vi "DunkFlips.vi"() -> ()   [LabVIEW 2015]
uses:
  <vilib>/Platform/TimedLoop/XDataNode/timing_clust.ctl
  <vilib>/Platform/TimedLoop/XDataNode/nitl_modes.ctl
  <vilib>/Platform/TimedLoop/XDataNode/wakeup.ctl
  <vilib>/rvi/Emulation/niFpgaGetClockAttributes.vi
  <vilib>/rvi/Emulation/niFpgaSctlEmulationGetInTimedLoop.vi
  <vilib>/rvi/Emulation/niFpgaEmulationReportErrorSimple.vi
  <vilib>/rvi/DataTransferAndStorage/Container/Common/niFpgaContainerGetUniqueNameForEmu.vi
  <vilib>/rvi/DataTransferAndStorage/Container/Common/niFpgaContainerSetEmuInfo.vi
  <vilib>/rvi/eio/common/nirviEmuReportErrorAndStop.vi
  <vilib>/rvi/eio/common/nirviEmuTemplateMethod_errors.vi
  <vilib>/rvi/DataTransferAndStorage/Container/Common/niFpgaContainerExecOnDevCompGetState.vi
  <vilib>/rvi/Emulation/niFpgaEmulationIsFPGAContextNoSignature.vi
  <vilib>/rvi/errors/niFpgaSetErrorForExecOnDevCompSimple.vi
  <vilib>/rvi/FIFO/Fifo_Resource/nirvififoEmulationSetSize.vi
  <vilib>/rvi/FIFO/Fifo_Resource/nirviFifoEmulationQueueMgr.vi
  <instcachedir>/0/nirviFifoEmulationQueueMgr_E5CAEC123FF24DC58D834DCA3CDAA9B5.lvgen/nirviFifoEmulationQueueMgr_E5CAEC123FF24DC58D834DCA3CDAA9B5_001.vi
  <vilib>/rvi/FIFO/Fifo_Resource/nirvififoEmulationDetermineInputValidOut.vi
  <vilib>/rvi/FIFO/Fifo_Resource/nirvififoEmulationCreateLock.vi
  <vilib>/rvi/Emulation/niFpgaProcessEmulError.vi
  <vilib>/rvi/FIFO/Fifo_Resource/nirvififoEmulationObtainLock.vi
  <vilib>/rvi/FIFO/Fifo_Resource/nirvififoEmulationReleaseLock.vi
  <vilib>/rvi/occurrence/nirviWaitOnOccurrenceBase.vi
  <vilib>/rvi/errors/nirviReportUnexpectedCaseInternalError.vi
  <vilib>/rvi/errors/nirviReportUnexpectedCaseInternalError (U32).vi
  <vilib>/Utility/error.llb/Clear Errors.vi
  <vilib>/rvi/interface/RandomDataEmulation/niFpgaRandomDataHandleErrors.vi
  <vilib>/rvi/Emulation/niFpgaCriticalErrorInLSC.vi
  <vilib>/rvi/Analysis/common/codeGenErrors/XNode/niFpgaXNodeCodeGenErrorHandle.vi
  <vilib>/rvi/Analysis/utilities/niFPGA Threshold Crossing Logic.vi
  <instcachedir>/0/nirviFifoEmulationQueueMgr_E5CAEC123FF24DC58D834DCA3CDAA9B5.lvgen/nirviFifoEmulationQueueMgr_E5CAEC123FF24DC58D834DCA3CDAA9B5_004.vi
  <instcachedir>/0/nirviFifoEmulationQueueMgr_E5CAEC123FF24DC58D834DCA3CDAA9B5.lvgen/nirviFifoEmulationQueueMgr_E5CAEC123FF24DC58D834DCA3CDAA9B5_000.vi
  <vilib>/rvi/LocalResourceManager/LocalResourceManager.xnode
  <vilib>/eio/EIONode/EIONode.xnode
  <vilib>/rvi/DataTransferAndStorage/Container/XNode/niFpgaContainer.xnode
  <vilib>/rvi/FIFO/Fifo_Resource/niFpgaFifoEmulationRefIn.vi
  <vilib>/rvi/Analysis/measure/period/templates/niFPGA Period Edge Direction.ctl
  <vilib>/rvi/Analysis/measure/butterworth/XNode/niFpgaButterworthFilter.xnode
  <vilib>/rvi/Analysis/measure/period/XNode/niFpgaAnalogPeriod.xnode
  <vilib>/Platform/TimedLoop/XDataNode/XDataNode.xnode
  <vilib>/rvi/FXPMathLib/basic elements/FxpDiscreteDelay/XNode/nifxpmath_DiscreteDelay.xnode
  <vilib>/rvi/interface/RandomDataEmulation/nirviRandomDataFpgaReadWriteTemplate.vi
  <vilib>/Platform/TimedLoop/XDataNode/XDNodeRunTimeDep.lvlib
panel:
  out "Time":i64=15
  out "TDOA 3":i64
  out "TDOA 2":i64
  out "TDOA 1":i64
  out "Period 4":u32=17
  out "Period 3":u32=15
  out "Period 1":u32=14
  out "Period 2":u32=30
  out "Boolean 4":bool
  out "Boolean 3":bool
  out "Boolean 2":bool
  out "Boolean":bool
  out "unsigned value":u16=109
  out "byte value":u16
  out "qfgLO!":i16=109
  in  "Baud Rate":u32=9600
  out "Real Baud Rate":u32=4167
  out "Des BABaus":u32=4167
  out "DIO Max":u16=18
  out "DIO Min":u16=15
  in  "FIFO Signal":u32
  out "Output 3":i64
  in  "High Pass":bool=TRUE
  in  "Low Pass":bool=TRUE
  in  "Hysteresis 4":fxp<+,16,2>
  in  "Hysteresis 3":fxp<+,16,2>
  in  "Hysteresis 2":fxp<+,16,2>
  out "Actual Sample Period Process (ticks)":u32=80
  in  "Min signal time gap (samples)":u32=500000
  in  "Min Amplitude 1":fxp<+/-,16,3>=0.0050048828125
  out "Output 1":i64
  out "AI0":sgl(slide)=-0.00048828125 scale=-10.0..10.0
  in  "Min Amplitude 2":fxp<+/-,16,3>=0.0050048828125
  out "Output 2":i64
  out "AI1":sgl(slide) scale=-10.0..10.0
  in  "Min Amplitude 3":fxp<+/-,16,3>=0.0050048828125
  out "AI2":sgl(slide)=-0.00048828125 scale=-10.0..10.0
  out "Output 4":i64
  in  "Hysteresis 1":fxp<+,16,2>
  in  "Min Amplitude 4":fxp<+/-,16,3>=0.0050048828125
  out "AI3":sgl(slide)=0.00024414062 scale=-10.0..10.0
  in  "Requested Sample Period (ticks)":u32=80
  out "Actual Sample Period Wave (ticks)":u32=80
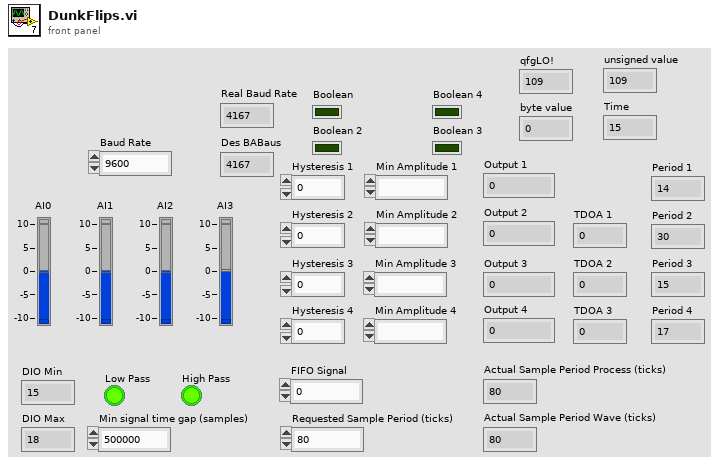
[diagram p1: front panel]
types:
  T1 = typedef "XDNodeRunTimeDep.lvlib/timing_clust.ctl" = cluster{"Expected End [f-1]":u64, "Actual End [f-1]":u64, "Finished Late? [f-1]":bool, "Expected End [i-1]":u64, "Actual End [i-1]":u64, "Finished Late? [i-1]":bool, "Expected Start [i]":u64, "Actual Start [i]":u64, "Expected Start [f]":u64, "Actual Start [f]":u64, "Source Name":string, "Structure Name":string, "Period":i64, "Deadline":i64, "Offset":i64, "Start":i64, "Priority":i32, "Timeout":i32, "Mode":T2, "Wakeup Reason":T3, "Error":errorcluster, "Source Type":string, "Secondary Source Type":string, "Global End Time":u64, "Global Start Time":u64, "Frame Duration":u64, "Iteration Duration":u64, "Assigned CPU":i32, "I/O Scan Engine Mode":u32}
  T2 = typedef "XDNodeRunTimeDep.lvlib/nitl_modes.ctl" = enum32{"No Change", "Process missed periods, maintain original phase", "Discard missed periods, maintain original phase", "Process missed periods, ignore original phase", "Discard missed periods, ignore original phase"}
  T3 = typedef "XDNodeRunTimeDep.lvlib/wakeup.ctl" = enum32{"Normal", "Aborted", "Asynchronous wakeup", "Timing source error", "Timed loop error", "Timeout"}
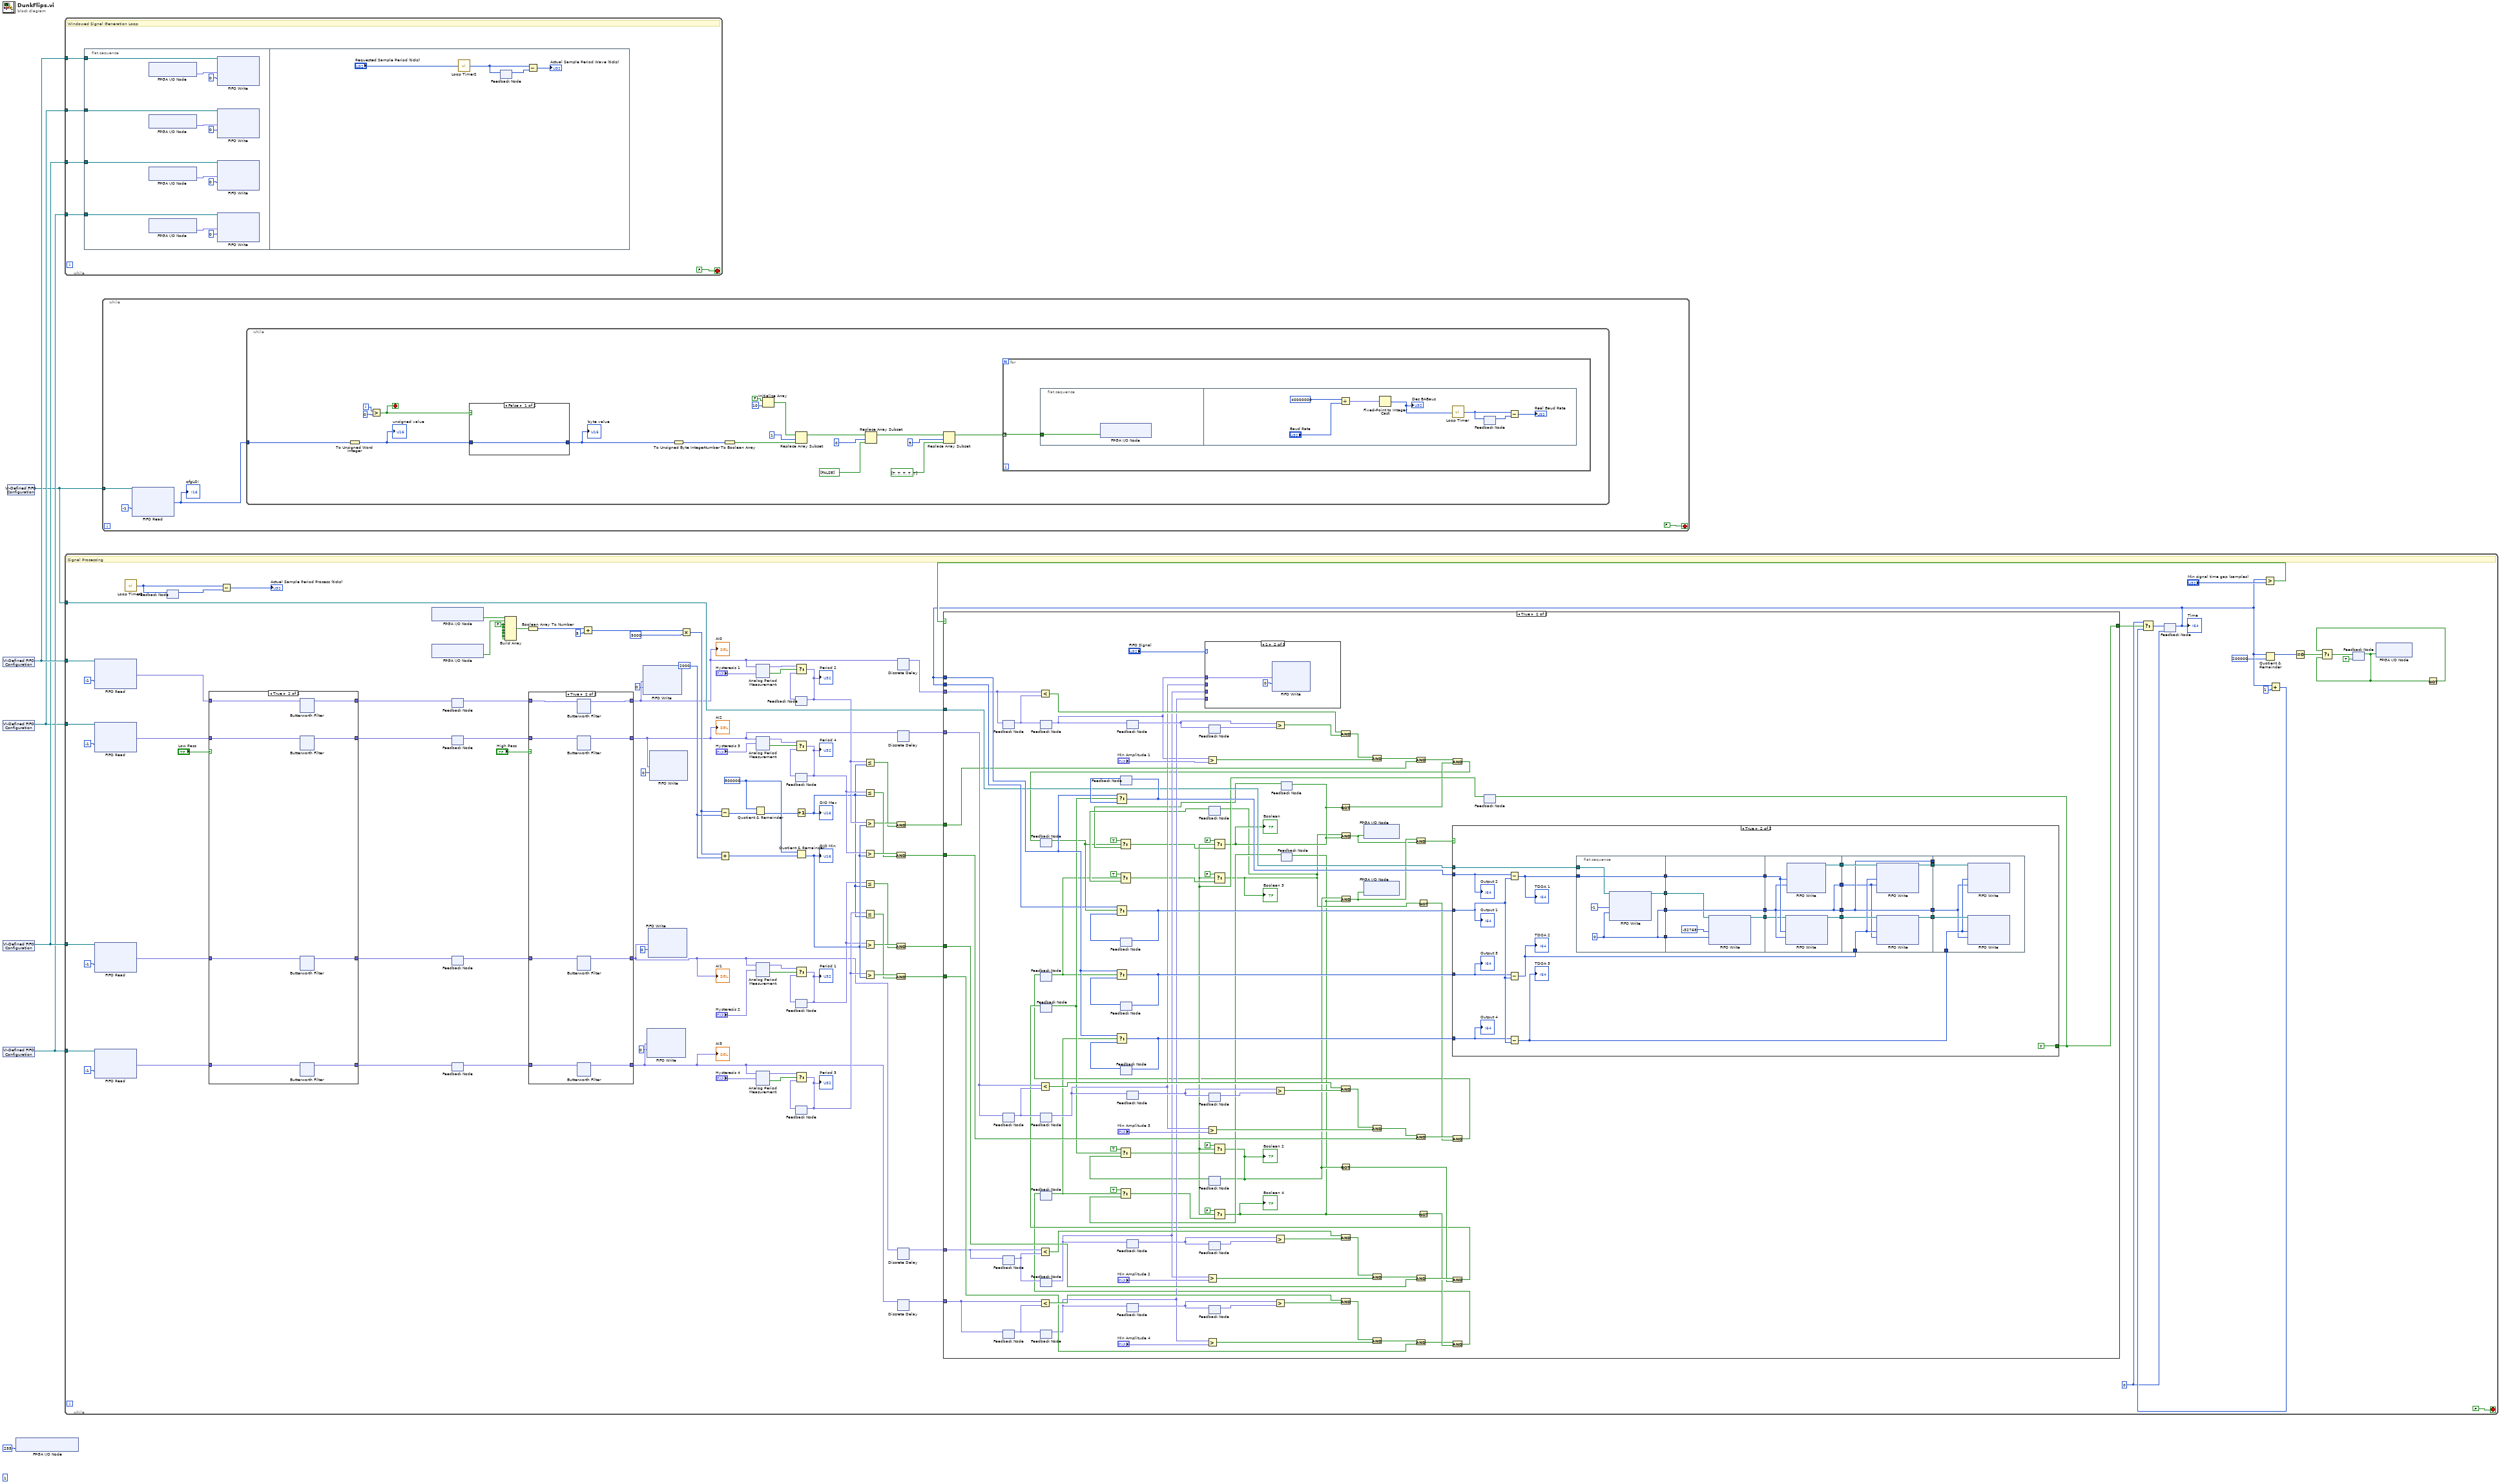
[diagram p0: block diagram]
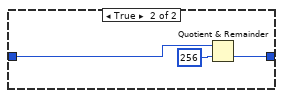
[diagram p2: hidden frame]
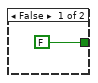
[diagram p5: hidden frame]
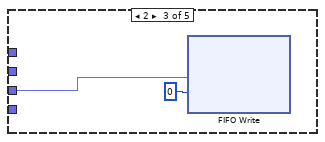
[diagram p7: hidden frame]
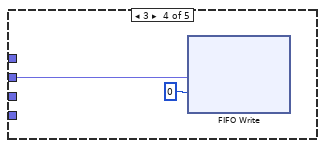
[diagram p8: hidden frame]
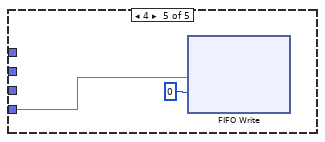
[diagram p9: hidden frame]
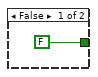
[diagram p10: hidden frame]
diagram:
  (unwired) 1 ("y")
  n1 = xnode "VI-Defined FIFO Configuration"() -> ("FIFO Out"=w6:refnum<k21>)
  n2 = xnode "VI-Defined FIFO Configuration"() -> ("FIFO Out"=w3:refnum<k21>)
  n3 = xnode "VI-Defined FIFO Configuration"() -> ("FIFO Out"=w5:refnum<k21>)
  n4 = xnode "VI-Defined FIFO Configuration"() -> ("FIFO Out"=w4:refnum<k21>)
  n5 = xnode "VI-Defined FIFO Configuration"() -> ("FIFO Out"=w2:refnum<k21>)
  n6 = xnode "FPGA I/O Node"("Connector3/DIOPORT0"=u8 255) -> ()  [unwired: 1 in, 1 out]
  n7 = while {
    tunnel: w6 -> [w11]
    tunnel: w5 -> [w9]
    tunnel: w3 -> [w8]
    tunnel: w4 -> [w7]
    stop <- FALSE stop-if-true
    # "Windowed Signal Generation Loop"
    n8 = flat-sequence {
      tunnel: w11 -> [w18]
      tunnel: w9 -> [w17]
      tunnel: w8 -> [w16]
      tunnel: w7 -> [w19]
      frame #0 {
        n9 = xnode "FPGA I/O Node"() -> ("Connector0/AI0"=w15:fxp<+/-,27,5>)  [unwired: 1 in, 1 out]
        n10 = xnode "FPGA I/O Node"() -> ("Connector0/AI2"=w13:fxp<+/-,27,5>)  [unwired: 1 in, 1 out]
        n11 = xnode "FPGA I/O Node"() -> ("Connector0/AI1"=w12:fxp<+/-,27,5>)  [unwired: 1 in, 1 out]
        n12 = xnode "FPGA I/O Node"() -> ("Connector0/AI3"=w14:fxp<+/-,27,5>)  [unwired: 1 in, 1 out]
        n13 = xnode ("FIFO Write")("Element"=w15, "Timeout"=0, "FIFO In"=w18) -> ()  [unwired: 2 out]
        n14 = xnode ("FIFO Write")("Element"=w13, "Timeout"=0, "FIFO In"=w16) -> ()  [unwired: 2 out]
        n15 = xnode ("FIFO Write")("Element"=w12, "Timeout"=0, "FIFO In"=w17) -> ()  [unwired: 2 out]
        n16 = xnode ("FIFO Write")("Element"=w14, "Timeout"=0, "FIFO In"=w19) -> ()  [unwired: 2 out]
      }
      frame #1 {
        n17 = call "Loop Timer2"("Count(Ticks)"="Requested Sample Period (ticks)") -> ("Tick Count(Ticks)"=w24:u32)
        n18 = feedback #1() -> (w25:u32)  [unwired: 1 in]
        n19 = feedback-in #1(w24) -> ()
        n20 = Subtract(x=w24, y=w25) -> (x-y=→"Actual Sample Period Wave (ticks)":u32)
      }
    }
  }
  n21 = while {
    tunnel: w6 -> [w111]
    tunnel: w5 -> [w112]
    tunnel: w3 -> [w110]
    tunnel: w4 -> [w124]
    tunnel: w2 -> [w70]
    stop <- FALSE stop-if-true
    w47 = i64 0
    w62 = u32 500000
    w66 = i16 2000
    w65 = FALSE
    # "Signal Processing"
    n22 = xnode ("FIFO Read")("Timeout"=i16 -1, "FIFO In"=w111) -> ("Element"=w90:fxp<+/-,16,4>)  [unwired: 2 out]
    n23 = xnode ("FIFO Read")("Timeout"=i16 -1, "FIFO In"=w110) -> ("Element"=w86:fxp<+/-,16,4>)  [unwired: 2 out]
    n24 = xnode ("FIFO Read")("Timeout"=i16 -1, "FIFO In"=w112) -> ("Element"=w89:fxp<+/-,16,4>)  [unwired: 2 out]
    n25 = xnode ("FIFO Read")("Timeout"=i16 -1, "FIFO In"=w124) -> ("Element"=w83:fxp<+/-,16,4>)  [unwired: 2 out]
    n26 = call "Loop Timer3"() -> ("Tick Count(Ticks)"=w103:u32)  [unwired: 1 in]
    n27 = feedback #2() -> (w104:u32)  [unwired: 1 in]
    n28 = feedback-in #2(w103) -> ()
    n29 = case shown="True" "Low Pass" {
      tunnel: [w173 w181] -> w91
      tunnel: w90 -> [w173 w180]
      tunnel: w89 -> [w172 w179]
      tunnel: [w172 w178] -> w88
      tunnel: w86 -> [w170 w177]
      tunnel: [w170 w176] -> w85
      tunnel: w83 -> [w171 w175]
      tunnel: [w171 w174] -> w82
      frame False {
      }
      frame True {
        n30 = xnode "Butterworth Filter"("input data"=w180) -> ("output data"=w181:fxp<+/-,20,8>)  [unwired: 2 in]
        n31 = xnode "Butterworth Filter"("input data"=w177) -> ("output data"=w176:fxp<+/-,20,8>)  [unwired: 2 in]
        n32 = xnode "Butterworth Filter"("input data"=w179) -> ("output data"=w178:fxp<+/-,20,8>)  [unwired: 2 in]
        n33 = xnode "Butterworth Filter"("input data"=w175) -> ("output data"=w174:fxp<+/-,20,8>)  [unwired: 2 in]
      }
    }
    n34 = Subtract(x=w103, y=w104) -> (x-y=→"Actual Sample Period Process (ticks)":u32)
    n35 = xnode "FPGA I/O Node"() -> ("Connector2/DIO0"=w69:bool)  [unwired: 1 in, 1 out]
    n36 = xnode "FPGA I/O Node"() -> ("Connector2/DIO1"=w68:bool)  [unwired: 1 in, 1 out]
    n37 = feedback #3() -> (w92:fxp<+/-,20,8>)  [unwired: 1 in]
    n38 = feedback-in #3(w91) -> ()
    n39 = feedback #4() -> (w84:fxp<+/-,20,8>)  [unwired: 1 in]
    n40 = feedback-in #4(w85) -> ()
    n41 = feedback #5() -> (w87:fxp<+/-,20,8>)  [unwired: 1 in]
    n42 = feedback-in #5(w88) -> ()
    n43 = feedback #6() -> (w81:fxp<+/-,20,8>)  [unwired: 1 in]
    n44 = feedback-in #6(w82) -> ()
    n45 = Build Array(w69, w68, w65, w65, w65, w65, w65, w65) -> (w67:bool[])
    n46 = Boolean Array To Number(Boolean array=w67) -> (number=w64:u8)
    n47 = case shown="True" "High Pass" {
      tunnel: w92 -> [w133 w141]
      tunnel: [w133 w140] -> w35
      tunnel: w87 -> [w132 w139]
      tunnel: w84 -> [w131 w138]
      tunnel: w81 -> [w130 w137]
      tunnel: [w132 w136] -> w31
      tunnel: [w131 w135] -> w33
      tunnel: [w130 w134] -> w29
      frame False {
      }
      frame True {
        n48 = xnode "Butterworth Filter"("input data"=w141) -> ("output data"=w140:fxp<+/-,24,12>)  [unwired: 2 in]
        n49 = xnode "Butterworth Filter"("input data"=w138) -> ("output data"=w135:fxp<+/-,24,12>)  [unwired: 2 in]
        n50 = xnode "Butterworth Filter"("input data"=w139) -> ("output data"=w136:fxp<+/-,24,12>)  [unwired: 2 in]
        n51 = xnode "Butterworth Filter"("input data"=w137) -> ("output data"=w134:fxp<+/-,24,12>)  [unwired: 2 in]
      }
    }
    "AI3" <- w29
    "AI2" <- w33
    "AI1" <- w31
    "AI0" <- w35
    n52 = Add(x=w64, y=i16 5) -> (x+y=w73:i16)
    n53 = xnode "FIFO Write"("Element"=w35, "Timeout"=0) -> ()  [unwired: 1 in, 2 out]
    n54 = xnode "FIFO Write"("Element"=w29, "Timeout"=0) -> ()  [unwired: 1 in, 2 out]
    n55 = xnode "FIFO Write"("Element"=w31, "Timeout"=0) -> ()  [unwired: 1 in, 2 out]
    n56 = xnode "FIFO Write"("Element"=w33, "Timeout"=0) -> ()  [unwired: 1 in, 2 out]
    n57 = Multiply(x=w73, y=i16 5000) -> (x*y=w72:u16)
    n58 = Subtract(x=w72, y=w66) -> (x-y=w61:u16)
    n59 = Add(x=w72, y=w66) -> (x+y=w63:u16)
    n60 = Quotient & Remainder(x=w62, y=w61) -> (floor(x/y)=w50:u32)  [unwired: 1 out]
    n61 = xnode "Analog Period Measurement"("input data"=w35, "direction"="Hysteresis 1") -> ("period (samples)"=w60:fxp<+,32,16>, "output valid"=w113:bool)  [unwired: 3 in, 2 out]
    n62 = xnode "Analog Period Measurement"("input data"=w33, "hysteresis"="Hysteresis 3") -> ("period (samples)"=w57:fxp<+,32,16>, "output valid"=w119:bool)  [unwired: 3 in, 2 out]
    n63 = xnode "Analog Period Measurement"("input data"=w31, "hysteresis"="Hysteresis 2") -> ("period (samples)"=w59:fxp<+,32,16>, "output valid"=w116:bool)  [unwired: 3 in, 2 out]
    n64 = xnode "Analog Period Measurement"("input data"=w29, "hysteresis"="Hysteresis 4") -> ("period (samples)"=w58:fxp<+,32,16>, "output valid"=w126:bool)  [unwired: 3 in, 2 out]
    n65 = feedback #7() -> (w102:fxp<+,32,16>)  [unwired: 1 in]
    n66 = Select(t=w60, s=w113, f=w102) -> (s? t:f=w53:fxp<+,32,16>)
    "Period 2" <- w53
    n67 = feedback-in #7(w53) -> ()
    n68 = feedback #8() -> (w100:fxp<+,32,16>)  [unwired: 1 in]
    n69 = Select(t=w57, s=w119, f=w100) -> (s? t:f=w55:fxp<+,32,16>)
    "Period 4" <- w55
    n70 = feedback-in #8(w55) -> ()
    n71 = Increment(x=w50) -> (x+1=w51:u32)
    "DIO Max" <- w51
    n72 = Quotient & Remainder(x=w62, y=w63) -> (floor(x/y)=w56:u32)  [unwired: 1 out]
    "DIO Min" <- w56
    n73 = feedback #9() -> (w101:fxp<+,32,16>)  [unwired: 1 in]
    n74 = Select(t=w59, s=w116, f=w101) -> (s? t:f=w52:fxp<+,32,16>)
    "Period 1" <- w52
    n75 = feedback-in #9(w52) -> ()
    n76 = feedback #10() -> (w99:fxp<+,32,16>)  [unwired: 1 in]
    n77 = Select(t=w58, s=w126, f=w99) -> (s? t:f=w54:fxp<+,32,16>)
    "Period 3" <- w54
    n78 = feedback-in #10(w54) -> ()
    n79 = Less Or Equal?(x=w53, y=w51) -> (x <= y?=w114:bool)
    n80 = Less Or Equal?(x=w55, y=w51) -> (x <= y?=w121:bool)
    n81 = Greater?(x=w53, y=w56) -> (0:w115:bool)
    n82 = Greater?(x=w55, y=w56) -> (0:w122:bool)
    n83 = Less Or Equal?(x=w52, y=w51) -> (x <= y?=w117:bool)
    n84 = Less Or Equal?(x=w54, y=w51) -> (x <= y?=w127:bool)
    n85 = Greater?(x=w52, y=w56) -> (0:w118:bool)
    n86 = Greater?(x=w54, y=w56) -> (0:w128:bool)
    n87 = And(x=w115, y=w114) -> (x .and. y?=w75:bool)
    n88 = And(x=w122, y=w121) -> (x .and. y?=w123:bool)
    n89 = And(x=w118, y=w117) -> (x .and. y?=w78:bool)
    n90 = And(x=w128, y=w127) -> (x .and. y?=w79:bool)
    n91 = xnode ("Discrete Delay")("D"=w35) -> ("Q"=w76:fxp<+/-,24,12>)
    n92 = xnode ("Discrete Delay")("D"=w33) -> ("Q"=w120:fxp<+/-,24,12>)
    n93 = xnode ("Discrete Delay")("D"=w31) -> ("Q"=w77:fxp<+/-,24,12>)
    n94 = xnode ("Discrete Delay")("D"=w29) -> ("Q"=w80:fxp<+/-,24,12>)
    n95 = feedback #11(w47) -> (w43:i64)
    "Time" <- w43
    n96 = Greater?(x=w43, y="Min signal time gap (samples)") -> (0:w109:bool)
    n97 = case shown="True" w109 {
      tunnel: w43 -> [_ w514]
      tunnel: w120 -> [_ w542]
      tunnel: w123 -> [_ w540]
      tunnel: w80 -> [_ w527]
      tunnel: w79 -> [_ w526]
      tunnel: w78 -> [_ w513]
      tunnel: w77 -> [_ w512]
      tunnel: w43 -> [_ w501]
      tunnel: w76 -> [_ w500]
      tunnel: w75 -> [_ w499]
      tunnel: w70 -> [_ w489]
      tunnel: [FALSE w488] -> w45
      frame False {
      }
      frame True {
        n98 = feedback #12() -> (w504:fxp<+/-,24,12>)  [unwired: 1 in]
        n99 = feedback-in #12(w500) -> ()
        n100 = feedback #13() -> (w547:fxp<+/-,24,12>)  [unwired: 1 in]
        n101 = feedback-in #13(w542) -> ()
        n102 = feedback #14() -> (w517:fxp<+/-,24,12>)  [unwired: 1 in]
        n103 = feedback-in #14(w512) -> ()
        n104 = feedback #15() -> (w530:fxp<+/-,24,12>)  [unwired: 1 in]
        n105 = feedback-in #15(w527) -> ()
        n106 = Less?(x=w500, y=w504) -> (x < y?=w511:bool)
        n107 = Less?(x=w542, y=w547) -> (x < y?=w538:bool)
        n108 = Less?(x=w512, y=w517) -> (x < y?=w524:bool)
        n109 = Less?(x=w527, y=w530) -> (x < y?=w537:bool)
        n110 = feedback #16() -> (w491:fxp<+/-,24,12>)  [unwired: 1 in]
        n111 = feedback-in #16(w504) -> ()
        n112 = feedback #17() -> (w459:bool)  [unwired: 1 in]
        n113 = feedback #18() -> (w454:bool)  [unwired: 1 in]
        n114 = feedback #19() -> (w464:bool)  [unwired: 1 in]
        n115 = feedback #20() -> (w493:fxp<+/-,24,12>)  [unwired: 1 in]
        n116 = feedback-in #20(w547) -> ()
        n117 = feedback #21() -> (w449:bool)  [unwired: 1 in]
        n118 = feedback #22() -> (w490:fxp<+/-,24,12>)  [unwired: 1 in]
        n119 = feedback-in #22(w517) -> ()
        n120 = feedback #23() -> (w492:fxp<+/-,24,12>)  [unwired: 1 in]
        n121 = feedback-in #23(w530) -> ()
        n122 = feedback #24() -> (w522:i64)  [unwired: 1 in]
        n123 = Select(t=w514, s=w464, f=w522) -> (s? t:f=w521:i64)
        n124 = feedback-in #24(w521) -> ()
        n125 = feedback #25() -> (w508:i64)  [unwired: 1 in]
        n126 = Select(t=w501, s=w459, f=w508) -> (s? t:f=w498:i64)
        n127 = feedback-in #25(w498) -> ()
        n128 = feedback #26() -> (w543:i64)  [unwired: 1 in]
        n129 = Select(t=w514, s=w454, f=w543) -> (s? t:f=w497:i64)
        n130 = feedback-in #26(w497) -> ()
        n131 = feedback #27() -> (w534:i64)  [unwired: 1 in]
        n132 = Select(t=w514, s=w449, f=w534) -> (s? t:f=w496:i64)
        n133 = feedback-in #27(w496) -> ()
        n134 = feedback #28() -> (w503:fxp<+/-,24,12>)  [unwired: 1 in]
        n135 = feedback-in #28(w491) -> ()
        n136 = feedback #29() -> (w548:fxp<+/-,24,12>)  [unwired: 1 in]
        n137 = feedback-in #29(w493) -> ()
        n138 = feedback #30() -> (w516:fxp<+/-,24,12>)  [unwired: 1 in]
        n139 = feedback-in #30(w490) -> ()
        n140 = feedback #31() -> (w529:fxp<+/-,24,12>)  [unwired: 1 in]
        n141 = feedback-in #31(w492) -> ()
        n142 = case shown="1" "FIFO Signal" {
          tunnel: w493 -> [_ _ _ w555 _]
          tunnel: w492 -> [_ _ _ _ w557]
          tunnel: w491 -> [_ w551 _ _ _]
          tunnel: w490 -> [_ _ w553 _ _]
          frame 0, Default {
          }
          frame 1 {
            n143 = xnode ("FIFO Write")("Element"=w551, "Timeout"=i16 0) -> ()  [unwired: 1 in, 2 out]
          }
          frame 2 {
            n144 = xnode ("FIFO Write")("Element"=w553, "Timeout"=i16 0) -> ()  [unwired: 1 in, 2 out]
          }
          frame 3 {
            n145 = xnode ("FIFO Write")("Element"=w555, "Timeout"=i16 0) -> ()  [unwired: 1 in, 2 out]
          }
          frame 4 {
            n146 = xnode ("FIFO Write")("Element"=w557, "Timeout"=i16 0) -> ()  [unwired: 1 in, 2 out]
          }
        }
        n147 = Greater?(x=w491, y="Min Amplitude 1") -> (0:w507:bool)
        n148 = Greater?(x=w493, y="Min Amplitude 3") -> (0:w544:bool)
        n149 = Greater?(x=w490, y="Min Amplitude 2") -> (0:w520:bool)
        n150 = Greater?(x=w492, y="Min Amplitude 4") -> (0:w533:bool)
        n151 = feedback #32() -> (w502:fxp<+/-,24,12>)  [unwired: 1 in]
        n152 = feedback-in #32(w503) -> ()
        n153 = feedback #33() -> (w474:bool)  [unwired: 1 in]
        n154 = Select(t=TRUE, s=w454, f=w474) -> (s? t:f=w472:bool)
        n155 = feedback #34() -> (w549:fxp<+/-,24,12>)  [unwired: 1 in]
        n156 = feedback-in #34(w548) -> ()
        n157 = feedback #35() -> (w484:bool)  [unwired: 1 in]
        n158 = Select(t=TRUE, s=w464, f=w484) -> (s? t:f=w483:bool)
        n159 = feedback #36() -> (w515:fxp<+/-,24,12>)  [unwired: 1 in]
        n160 = feedback-in #36(w516) -> ()
        n161 = feedback #37() -> (w528:fxp<+/-,24,12>)  [unwired: 1 in]
        n162 = feedback-in #37(w529) -> ()
        n163 = Greater?(x=w503, y=w502) -> (0:w510:bool)
        n164 = Greater?(x=w548, y=w549) -> (0:w539:bool)
        n165 = Greater?(x=w516, y=w515) -> (0:w525:bool)
        n166 = Greater?(x=w529, y=w528) -> (0:w536:bool)
        n167 = feedback #38() -> (w469:bool)  [unwired: 1 in]
        n168 = Select(t=TRUE, s=w459, f=w469) -> (s? t:f=w471:bool)
        n169 = feedback #39() -> (w479:bool)  [unwired: 1 in]
        n170 = Select(t=TRUE, s=w449, f=w479) -> (s? t:f=w481:bool)
        n171 = And(x=w511, y=w510) -> (x .and. y?=w506:bool)
        n172 = And(x=w538, y=w539) -> (x .and. y?=w545:bool)
        n173 = And(x=w524, y=w525) -> (x .and. y?=w519:bool)
        n174 = And(x=w537, y=w536) -> (x .and. y?=w532:bool)
        n175 = And(x=w506, y=w507) -> (x .and. y?=w509:bool)
        n176 = And(x=w545, y=w544) -> (x .and. y?=w541:bool)
        n177 = And(x=w519, y=w520) -> (x .and. y?=w523:bool)
        n178 = And(x=w532, y=w533) -> (x .and. y?=w535:bool)
        n179 = And(x=w509, y=w499) -> (x .and. y?=w463:bool)
        n180 = And(x=w541, y=w540) -> (x .and. y?=w458:bool)
        n181 = And(x=w523, y=w513) -> (x .and. y?=w468:bool)
        n182 = And(x=w535, y=w526) -> (x .and. y?=w452:bool)
        n183 = feedback #40() -> (w470:bool)  [unwired: 1 in]
        n184 = Select(t=FALSE, s=w470, f=w471) -> (s? t:f=w461:bool)
        "Boolean" <- w461
        n185 = Select(t=FALSE, s=w470, f=w472) -> (s? t:f=w456:bool)
        "Boolean 3" <- w456
        n186 = feedback-in #33(w456) -> ()
        n187 = Select(t=FALSE, s=w470, f=w483) -> (s? t:f=w466:bool)
        "Boolean 2" <- w466
        n188 = feedback-in #35(w466) -> ()
        n189 = Select(t=FALSE, s=w470, f=w481) -> (s? t:f=w451:bool)
        "Boolean 4" <- w451
        n190 = feedback-in #38(w461) -> ()
        n191 = feedback-in #39(w451) -> ()
        n192 = Not(x=w461) -> (.not. x?=w462:bool)
        n193 = Not(x=w466) -> (.not. x?=w467:bool)
        n194 = And(x=w456, y=w461) -> (x .and. y?=w486:bool)
        n195 = And(x=w466, y=w451) -> (x .and. y?=w487:bool)
        n196 = xnode "FPGA I/O Node"("User LED2"=w486) -> ()  [unwired: 1 in, 1 out]
        n197 = xnode "FPGA I/O Node"("User LED1"=w487) -> ()  [unwired: 1 in, 1 out]
        n198 = And(x=w487, y=w486) -> (x .and. y?=w495:bool)
        n199 = Not(x=w456) -> (.not. x?=w457:bool)
        n200 = Not(x=w451) -> (.not. x?=w453:bool)
        n201 = And(x=w463, y=w462) -> (x .and. y?=w460:bool)
        n202 = feedback-in #17(w460) -> ()
        n203 = And(x=w458, y=w457) -> (x .and. y?=w455:bool)
        n204 = feedback-in #18(w455) -> ()
        n205 = And(x=w468, y=w467) -> (x .and. y?=w465:bool)
        n206 = feedback-in #19(w465) -> ()
        n207 = And(x=w452, y=w453) -> (x .and. y?=w450:bool)
        n208 = feedback-in #21(w450) -> ()
        n209 = case shown="True" w495 {
          tunnel: w521 -> [_ w572]
          tunnel: w498 -> [_ w575]
          tunnel: w497 -> [_ w573]
          tunnel: w496 -> [_ w574]
          tunnel: [FALSE TRUE] -> w488
          tunnel: w489 -> [_ w569]
          frame False {
          }
          frame True {
            n210 = Subtract(x=w572, y=w575) -> (x-y=w561:i64)
            "TDOA 1" <- w561
            n211 = Subtract(x=w573, y=w575) -> (x-y=w560:i64)
            "TDOA 2" <- w560
            n212 = Subtract(x=w574, y=w575) -> (x-y=w559:i64)
            "TDOA 3" <- w559
            n213 = flat-sequence {
              tunnel: w561 -> [w587]
              tunnel: [w587] -> w568
              tunnel: [w583] -> w566
              tunnel: w569 -> [w585]
              tunnel: [w584] -> w564
              tunnel: [w583] -> w562
              tunnel: w568 -> [w593]
              tunnel: [w593] -> w567
              tunnel: w566 -> [w592]
              tunnel: [w592] -> w565
              tunnel: w564 -> [w591]
              tunnel: [w590] -> w563
              tunnel: w562 -> [w589]
              tunnel: [w598] -> w581
              tunnel: [w595] -> w579
              tunnel: [w595] -> w577
              tunnel: [w597] -> w571
              tunnel: w567 -> [w596]
              tunnel: w565 -> [w595]
              tunnel: w563 -> [w594]
              tunnel: w581 -> [w605]
              tunnel: [w604] -> w580
              tunnel: w579 -> [w599]
              tunnel: [w603] -> w578
              tunnel: w577 -> [w603]
              tunnel: [w603] -> w576
              tunnel: w560 -> [w600]
              tunnel: w571 -> [w602]
              tunnel: [w601] -> w570
              tunnel: w580 -> [w609]
              tunnel: w578 -> [w606]
              tunnel: w576 -> [_]
              tunnel: w559 -> [w607]
              tunnel: w570 -> [w608]
              frame #0 {
                w583 = i16 0
                n214 = xnode ("FIFO Write")("Element"=i16 -1, "Timeout"=w583, "FIFO In"=w585) -> ("FIFO Out"=w584:refnum<k21>)  [unwired: 1 out]
              }
              frame #1 {
                n215 = xnode ("FIFO Write")("Element"=i16 -32768, "Timeout"=w589, "FIFO In"=w591) -> ("FIFO Out"=w590:refnum<k21>)  [unwired: 1 out]
              }
              frame #2 {
                n216 = xnode ("FIFO Write")("Element"=w596, "Timeout"=w595, "FIFO In"=w594) -> ("FIFO Out"=w597:refnum<k21>)  [unwired: 1 out]
                n217 = xnode ("FIFO Write")("Element"=w596, "Timeout"=w595) -> ("FIFO Out"=w598:refnum<k21>)  [unwired: 1 in, 1 out]
              }
              frame #3 {
                n218 = xnode ("FIFO Write")("Element"=w600, "Timeout"=w599, "FIFO In"=w605) -> ("FIFO Out"=w604:refnum<k21>)  [unwired: 1 out]
                n219 = xnode ("FIFO Write")("Element"=w600, "Timeout"=w599, "FIFO In"=w602) -> ("FIFO Out"=w601:refnum<k21>)  [unwired: 1 out]
              }
              frame #4 {
                n220 = xnode ("FIFO Write")("Element"=w607, "Timeout"=w606, "FIFO In"=w609) -> ()  [unwired: 2 out]
                n221 = xnode ("FIFO Write")("Element"=w607, "Timeout"=w606, "FIFO In"=w608) -> ()  [unwired: 2 out]
              }
            }
            "Output 2" <- w572
            "Output 1" <- w575
            "Output 3" <- w573
            "Output 4" <- w574
          }
        }
        n222 = feedback-in #40(w488) -> ()
      }
    }
    n223 = Quotient & Remainder(x=w43, y=200000) -> (x-y*floor(x/y)=w41:i64)  [unwired: 1 out]
    n224 = Add(x=w43, y=i64 1) -> (x+y=w48:i64)
    n225 = Select(t=w47, s=w45, f=w48) -> (s? t:f=w46:i64)
    n226 = feedback-in #11(w46) -> ()
    n227 = Equal To 0?(x=w41) -> (x = 0?=w40:bool)
    n228 = feedback #41(TRUE) -> (w37:bool)
    n229 = xnode "FPGA I/O Node"("User LED3"=w37) -> ()  [unwired: 1 in, 1 out]
    n230 = Not(x=w37) -> (.not. x?=w38:bool)
    n231 = Select(t=w38, s=w40, f=w37) -> (s? t:f=w36:bool)
    n232 = feedback-in #41(w36) -> ()
  }
  n233 = while {
    tunnel: w2 -> [w847]
    stop <- FALSE stop-if-true
    n234 = xnode ("FIFO Read")("Timeout"=i16 -1, "FIFO In"=w847) -> ("Element"=w844:i16)  [unwired: 2 out]
    "qfgLO!" <- w844
    n235 = while {
      tunnel: w844 -> [w853]
      i -> [w851]
      stop <- w848 stop-if-true
      n236 = To Unsigned Word Integer(number=w853) -> (unsigned 16bit integer=w852:u16)
      "unsigned value" <- w852
      n237 = Greater?(x=w851, y=i16 0) -> (0:w848:bool)
      n238 = case shown="False" w848 {
        tunnel: [w867 w868] -> w850
        tunnel: w852 -> [w867 w870]
        frame False {
        }
        frame True {
          n239 = Quotient & Remainder(x=w870, y=u16 256) -> (floor(x/y)=w868:u16)  [unwired: 1 out]
        }
      }
      "byte value" <- w850
      n240 = To Unsigned Byte Integer(number=w850) -> (unsigned 8bit integer=w849:u8)
      n241 = Number To Boolean Array(number=w849) -> (Boolean array=w858:bool[])
      n242 = Initialize Array(FALSE, i16 10) -> (w856:bool[])
      n243 = Replace Array Subset(array=w856, new element=w858, index=1) -> (w859:bool[])
      n244 = Replace Array Subset(array=w859, new element=bool[] [FALSE], index=0) -> (w864:bool[])
      n245 = Replace Array Subset(array=w864, new element=bool[] [TRUE, TRUE, TRUE, TRUE, TRUE], index=9) -> (w865:bool[])
      n246 = for {
        tunnel: w865 -> [w871] mode=indexing
        n247 = flat-sequence {
          tunnel: w871 -> [w872]
          frame #0 {
            n248 = xnode "FPGA I/O Node"("Connector1/DIO0"=w872) -> ()  [unwired: 1 in, 1 out]
          }
          frame #1 {
            n249 = Divide(x=40000000, y="Baud Rate") -> (x/y=w874:fxp<+/-,16,16>)
            n250 = Fixed-Point to Integer Cast(1:w874) -> (0:w873:i16)
            "Des BABaus" <- w873
            n251 = call "Loop Timer"("Count(Ticks)"=w873) -> ("Tick Count(Ticks)"=w877:u32)
            n252 = feedback #42() -> (w878:u32)  [unwired: 1 in]
            n253 = feedback-in #42(w877) -> ()
            n254 = Subtract(x=w877, y=w878) -> (x-y=→"Real Baud Rate":u32)
          }
        }
      }
    }
  }
